vi "HapticSTM_Feedblackless_testdata_with_calibration.vi"() -> ()   [LabVIEW 2019]
uses:
  <vilib>/Analysis/3filter.llb/Filter Passband Type.ctl
  <vilib>/Utility/file.llb/Read Delimited Spreadsheet (DBL).vi
  <userlib>/HapticSTM/Feedbackless - Testdata/GlobalClicksHeight.vi
  <userlib>/HapticSTM/HapticSTM.lvlib
  <vilib>/ptbypt/NI_PtbyPt.lvlib
  <vilib>/Analysis/NI_AALBase.lvlib
  <userlib>/Calibration/Calibration.lvlib
panel:
  out "Button":bool
  out "Zpos":cluster{dbl, "Y":dbl, i16}(graph)
  out "Filtered Current":dbl
  in  "Reset Clicks":bool
  out "Scaled Force and Current":cluster{dbl, "Filtered x":dbl, dbl}(graph)
  in  "Maximum (pA)":dbl=9000.0
  in  "Setpoint (pA)":dbl=100.0
  out "PLANE HEIGHT":dbl
  out "Current":dbl
  out "Origin Y":dbl
  out "Origin X":dbl
  out "Output Z":dbl
  in  "Rough adjust":dbl
  out "Nano Z":dbl
  out "Width":dbl
  out "VY":dbl
  out "VZ":dbl
  out "VX":dbl
  in  "Drag":dbl=1.0
  in  "STOP":bool
  in  "START":bool
  out "Fy":dbl
  out "Fz":dbl
  out "phi":dbl
  out "psi":dbl
  out "Fx":dbl
  out "theta":dbl
  out "x":dbl
  out "y":dbl
  out "z":dbl
  in  "Fine adjust":dbl=3.5
  out "Clicks":dbl
  out "Height":dbl
  # "Sample Window"
  # "Position"
  # "Sensitivity"
  # "Force"
  # "STM I/O"
  # "Angles"
  # "Current"
  # "Velocity"
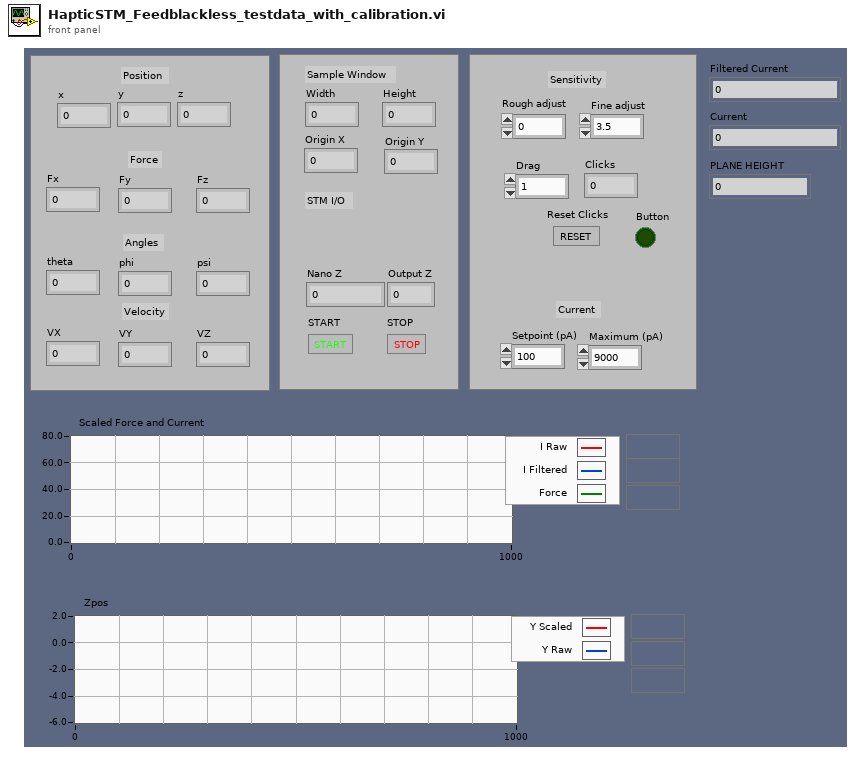
[diagram p1: front panel]
types:
  T1 = typedef "NI_AALBase.lvlib/Filter Passband Type.ctl" = enum32{"Lowpass", "Highpass", "Bandpass", "Bandstop"}
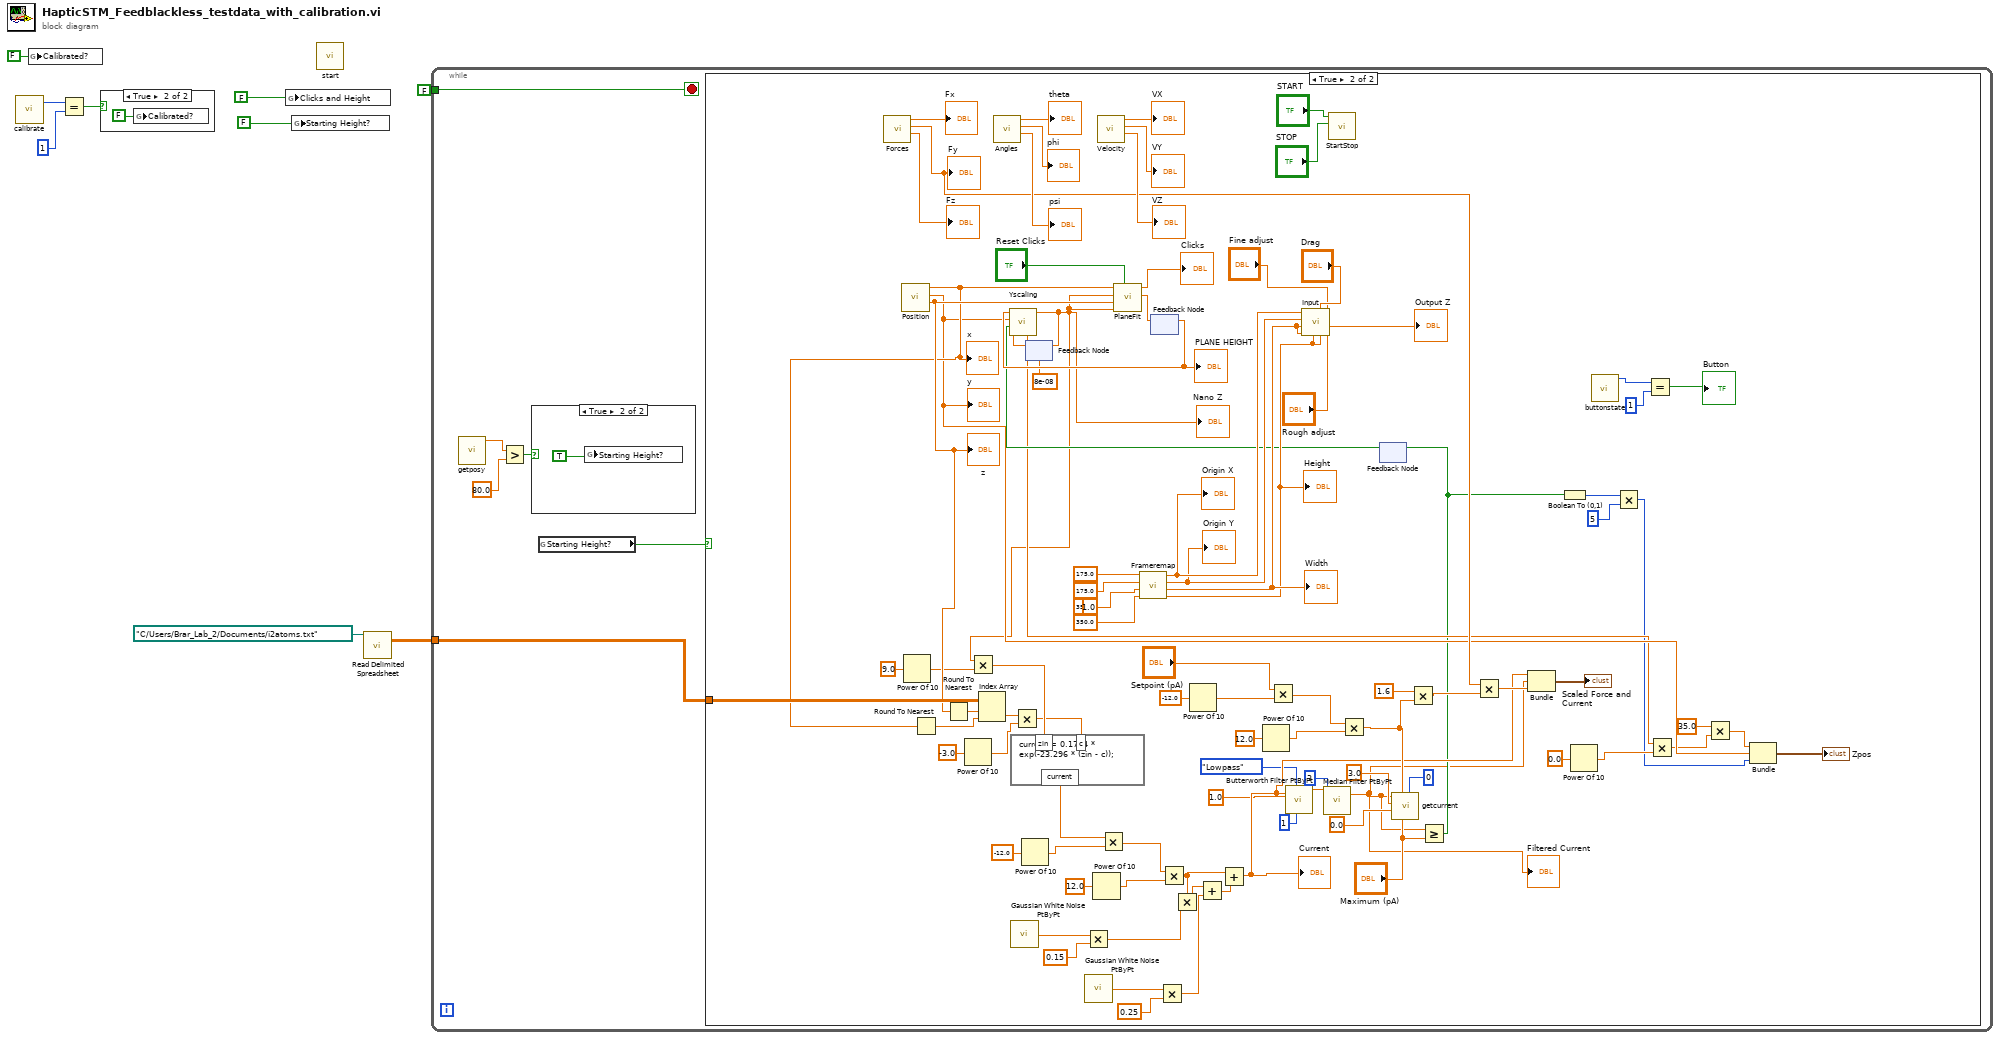
[diagram p0: block diagram]
diagram:
  n1 = call <userlib>:"calibrate.vi"() -> ("function return"=w3:i32)  [unwired: 11 in]
  n2 = global write "GlobalClicksHeight.vi" "Calibrated?"(FALSE ("Calibrated?")) -> ()
  n3 = Equal?(x=w3, y=1) -> (x = y?=w1:bool)
  n4 = case shown="True" w1 {
    frame False {
    }
    frame True {
      n5 = global write "GlobalClicksHeight.vi" "Calibrated?"(FALSE ("Calibrated?")) -> ()
    }
  }
  n6 = global write "GlobalClicksHeight.vi" "Clicks and Height"(FALSE ("Clicks and Height")) -> ()
  n7 = global write "GlobalClicksHeight.vi" "Starting Height?"(FALSE ("Clicks and Height")) -> ()
  n8 = call <userlib>:"start.vi"() -> ()  [unwired: 11 in, 1 out]
  n9 = call-poly <vilib>:"Read Delimited Spreadsheet.vi"("file path (dialog if empty)"=path "C:/Users/Brar_Lab_2/Documents/i2atoms.txt") -> ("all rows"=w8:dbl[][])  [unwired: 9 in, 5 out]
  n10 = while {
    tunnel: FALSE -> [w16]
    tunnel: w8 -> [w15]
    stop <- w16 stop-if-true
    n11 = call <userlib>:"getposy.vi"() -> ("function return"=w14:dbl)  [unwired: 11 in]
    n12 = Greater?(x=w14, y=80.0) -> (0:w12:bool)
    n13 = case shown="True" w12 {
      frame False {
      }
      frame True {
        n14 = global write "GlobalClicksHeight.vi" "Starting Height?"(TRUE ("Clicks and Height")) -> ()
      }
    }
    n15 = global read "GlobalClicksHeight.vi" "Starting Height?"() -> (w11:bool)
    n16 = case shown="True" w11 {
      tunnel: w15 -> [_ w72]
      frame False {
      }
      frame True {
        (unwired) 1.0 ("FO X")
        n17 = call <userlib>:"Forces.vi"() -> ("Fz"=→"Fz":dbl, "Fy"=w58:dbl, "Fx"=→"Fx":dbl)  [unwired: 9 in]
        "Fy" <- w58
        n18 = call <userlib>:"Position.vi"() -> ("Z"=w69:dbl, "Y"=w40:dbl, "X"=w68:dbl)  [unwired: 9 in]
        "x" <- w68
        "y" <- w40
        "z" <- w69
        n19 = Power Of 10(x=9.0) -> (10^x=w66:dbl)
        n20 = Round To Nearest(number=w68) -> (nearest integer value=w70:dbl)
        n21 = Round To Nearest(number=w69) -> (nearest integer value=w71:dbl)
        n22 = Power Of 10(x=-3.0) -> (10^x=w61:dbl)
        n23 = Index Array(array=w72, index (row)=w71, index (col)=w70) -> (element=w62:dbl)
        n24 = call <userlib>:"Angles.vi"() -> ("psi"=→"psi":dbl, "phi"=→"phi":dbl, "theta"=→"theta":dbl)  [unwired: 9 in]
        n25 = call <vilib>:"Gaussian White Noise PtByPt.vi"() -> ("Gaussian white noise"=w57:dbl)  [unwired: 3 in]
        n26 = Multiply(x=w62, y=w61) -> (x*y=w60:dbl)
        n27 = Power Of 10(x=-12.0) -> (10^x=w83:dbl)
        n28 = feedback #1(8e-08 ("y scaled")) -> (w21:dbl)
        n29 = Multiply(x=w57, y=0.15) -> (x*y=w55:dbl)
        n30 = call <vilib>:"Gaussian White Noise PtByPt.vi"() -> ("Gaussian white noise"=w52:dbl)  [unwired: 3 in]
        n31 = Power Of 10(x=12.0) -> (10^x=w92:dbl)
        n32 = call <userlib>:"Velocity.vi"() -> ("VZ"=→"VZ":dbl, "VY"=→"VY":dbl, "VX"=→"VX":dbl)  [unwired: 9 in]
        n33 = call <userlib>:"Frameremap.vi"("FH"=350.0 ("FO X"), "FW"=350.0 ("FO X"), "FO Z"=175.0 ("FO X"), "FO X"=175.0) -> ("FH"=w99:dbl, "FW"=w100:dbl, "Z Origin"=w84:dbl, "X Origin"=w85:dbl)  [unwired: 4 in]
        "Height" <- w99
        "Width" <- w100
        "Origin X" <- w85
        "Origin Y" <- w84
        n34 = feedback #2() -> (w86:dbl)  [unwired: 1 in]
        "PLANE HEIGHT" <- w86
        n35 = Multiply(x=w52, y=0.25) -> (x*y=w48:dbl)
        n36 = Power Of 10(x=-12.0) -> (10^x=w78:dbl)
        n37 = Power Of 10(x=12.0) -> (10^x=w80:dbl)
        n38 = Multiply(x="Setpoint (pA)", y=w78) -> (x*y=w76:dbl)
        n39 = call <userlib>:"Input.vi"("Current * 10^input"="Rough adjust", "Sensitivity"="Fine adjust", "Scopez"=w99, "Drag"="Drag", "FH"=w99, "FW"=w100, "Scopex"=w100, "Z origin"=w84, "X origin"=w85) -> ("Scaled Current"=→"Output Z":dbl)  [unwired: 2 in]
        n40 = call <userlib>:"StartStop.vi"("STOP"="STOP", "START"="START") -> ()  [unwired: 10 in]
        n41 = Multiply(x=w76, y=w80) -> (x*y=w45:dbl)
        n42 = feedback #3() -> (w74:bool)  [unwired: 1 in]
        n43 = call <userlib>:"Yscaling.vi"("Nano Z Read"=w21, "Current Maxed?"=w74, "Y"=w40, "Plane Height"=w86) -> ("y scaled"=w20:dbl, "Testoutput"=w36:dbl)  [unwired: 6 in]
        "Nano Z" <- w20
        n44 = Multiply(x=w20, y=w66) -> (x*y=w64:dbl)
        n45 = formula code="current = 0.1714 * exp(-23.296 * (zin - c));"("zin"=w64, "c"=w60) -> ("current"=w67:dbl)
        n46 = feedback-in #1(w20) -> ()
        n47 = Multiply(x=w67, y=w83) -> (x*y=w81:dbl)
        n48 = call <userlib>:"PlaneFit.vi"("Reset Clicks"="Reset Clicks", "Y PEN"=w20, "Z"=w69, "Nano Z"=w20, "X"=w68) -> ("Output"=w95:dbl, "Clicks"=→"Clicks":dbl)  [unwired: 5 in]
        n49 = feedback-in #2(w95) -> ()
        n50 = Multiply(x=w81, y=w92) -> (x*y=w54:dbl)
        n51 = Multiply(x=w54, y=w55) -> (x*y=w49:dbl)
        n52 = Add(x=w49, y=w48) -> (x+y=w50:dbl)
        n53 = Add(x=w54, y=w50) -> (x+y=w32:dbl)
        "Current" <- w32
        n54 = call <vilib>:"Butterworth Filter PtByPt.vi"("order"=1, "filter type"=Filter_Passband_Type."Lowpass", "sampling freq: fs"=1.0, "x"=w32) -> ("Filtered x"=w24:dbl)  [unwired: 5 in, 1 out]
        n55 = call <vilib>:"Median Filter PtByPt.vi"("rank"=3, "x"=w24) -> ("Filtered x"=w23:dbl)  [unwired: 2 in, 1 out]
        "Filtered Current" <- w23
        n56 = call <userlib>:"getcurrent.vi"("forcemode"=0, "maxcurrentin"="Maximum (pA)", "setpoint"=w45, "minforcey"=0.0, "maxforcey"=3.0, "currentin"=w23) -> ()  [unwired: 6 in]
        n57 = Multiply(x=1.6 ("y"), y=w45) -> (x*y=w46:dbl)
        n58 = Greater Or Equal?(x=w23, y="Maximum (pA)") -> (x >= y?=w29:bool)
        n59 = feedback-in #3(w29) -> ()
        n60 = Multiply(x=w58, y=w46) -> (x*y=w53:dbl)
        n61 = Bundle(w32, "Filtered x"=w23, w53) -> (→"Scaled Force and Current":cluster{dbl, "Filtered x":dbl, dbl})  [unwired: 1 in]
        n62 = Boolean To (0,1)(Boolean=w29) -> (0, 1=w28:i16)
        n63 = Power Of 10(x=0.0) -> (10^x=w43:dbl)
        n64 = call <userlib>:"buttonstate.vi"() -> ("function return"=w35:i32)  [unwired: 11 in]
        n65 = Multiply(x=w28, y=i16 5) -> (x*y=w26:i16)
        n66 = Equal?(x=w35, y=1) -> (x = y?=→"Button":bool)
        n67 = Multiply(x=w36, y=w43) -> (x*y=w38:dbl)
        n68 = Multiply(x=35.0, y=w38) -> (x*y=w39:dbl)
        n69 = Bundle(w39, "Y"=w40, w26) -> (→"Zpos":cluster{dbl, "Y":dbl, i16})  [unwired: 1 in]
      }
    }
  }
